vi "UDP Data Share Sender.vi"(6 "timeout ms (25000)":i32, 7 "Remote Port":u16=61557, 8 "error in (no error)":errorcluster, 9 "Exit?":bool, 10 "Data to send":string, 11 "Local Port":u16=61556) -> (0 "error out":errorcluster)   [LabVIEW 2011]
doc: "This VI is meant to be used in a LabVIEW VI that needs to send data to a web service VI or other VI that is not in this VIs application space. This is GLOBAL data that is updated on a regular basis.\n\n\nVersion 1.0 - 02/13/2013\n\nPhaeron, Inc.\nwww.phaeron.com\ninfo@phaeron.com"
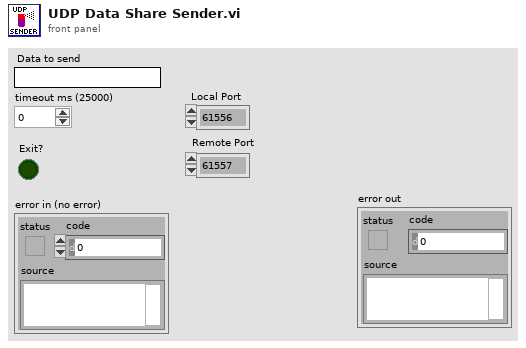
[diagram p1: front panel]
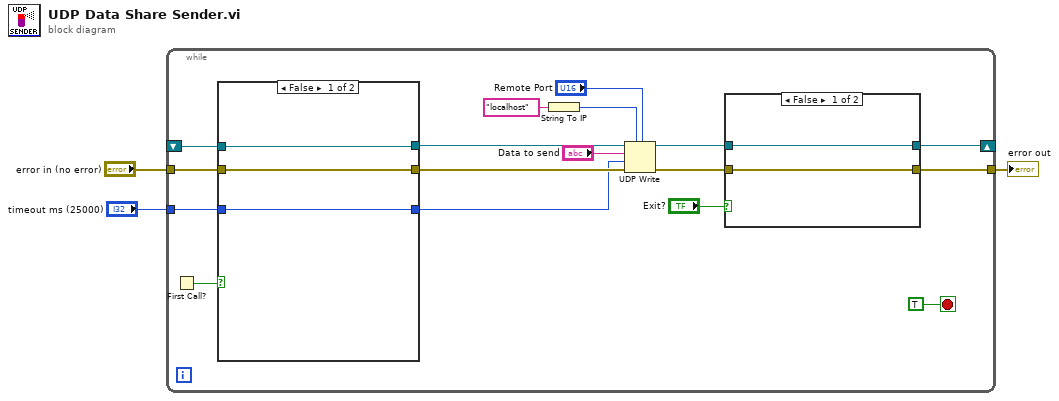
[diagram p0: block diagram]
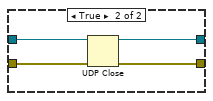
[diagram p2: hidden frame]
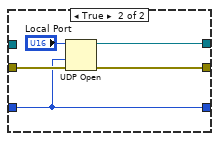
[diagram p3: hidden frame]
diagram:
  n1 = while {
    shift-right: [w6] -> _
    shift-left: _ -> [w19]
    tunnel: "error in (no error)" -> [w18]
    tunnel: "timeout ms (25000)" -> [w10]
    tunnel: [w5] -> w1
    stop <- TRUE stop-if-true
    n2 = First Call?() -> (First Call?: T/F=w20:bool)
    n3 = case shown="False" w20 {
      tunnel: w19 -> [w27 _]
      tunnel: w18 -> [w29 w33]
      tunnel: [w29 w32] -> w17
      tunnel: [w27 w31] -> w11
      tunnel: w10 -> [w28 w30]
      tunnel: [w28 w30] -> w9
      frame False {
      }
      frame True {
        n4 = UDP Open(8:w33, 9:w30, 11:"Local Port") -> (port=w31:refnum<k16>, 0:w32:errorcluster)  [unwired: 3 out]
      }
    }
    n5 = String To IP(1:"localhost" ("name")) -> (0:w15:u32)
    n6 = UDP Write(address=w15, port or service name="Remote Port", connection ID=w11, data in="Data to send", 8:w17, 9:w9) -> (error out=w8:errorcluster, 3:w7:refnum<k16>)
    n7 = case shown="False" "Exit?" {
      tunnel: w8 -> [w21 w26]
      tunnel: w7 -> [w22 w25]
      tunnel: [w22 w24] -> w6
      tunnel: [w21 w23] -> w5
      frame False {
      }
      frame True {
        n8 = UDP Close(connection ID=w25, 8:w26) -> (connection ID out=w24:refnum<k16>, error out=w23:errorcluster)
      }
    }
  }
  "error out" <- w1
